vi "Begin map measurement.vi"(8 "Sweep down\ntime [ms]":dbl=500.0 format="%#_13g", 9 "VID control":T4 {"Multip" items=["1"=1, "2"=2, "3"=3, "4"=4, "6"=6, "8"=8, "9"=9]; "AMC" items=["9"=9, "12"=12]}, 10 "Map parameters":T2={"B_start[T]"=0.0, "B_End[T]"=0.0, "B_rate [mT/s]"=0.0, "F_start[GHz]"=0.0, "F_end[GHz]"=0.0, "Sampling rate"=0, "Tmp [K]"=0.0, "Wait[min]"=0.0, "Points"=0, "Display signal"=enum."Phi", "Signal treat"=enum."None", "Sweep [s]"=2.0} {"Sampling rate" items=["117 ks/S"=9, "58.6 kS/s"=10, "29.3 kS/s"=11, "14.6 kS/s"=12, "7.32 kS/s"=13, "3.66 kS/s"=14, "1.83 kS/s"=15]}, 11 "Referencies in":T1) -> (0 "error out":errorcluster)   [LabVIEW 2022 SP3]
uses:
  Datatypes/THz parameters.ctl
  Datatypes/Map parameters.ctl
  Subsystem modules/Lock-in module/ctl/OSC sampling rate.ctl
  Subsystem modules/Messenger service/Data types/Messenger referencies.ctl
  Subsystem modules/Lock-in module/ctl/MFLI_message for module.ctl
  Subsystem modules/Lock-in module/ctl/MFLI_command enum.ctl
  Subsystem modules/THz module/ctl/THz Message for module.ctl
  Subsystem modules/THz module/ctl/THz commands enum.ctl
  Subsystem modules/THz module/ctl/THz sweep parameters.ctl
  Subsystem modules/Magnet module/ctl/MSG to magnet.ctl
  Subsystem modules/Magnet module/ctl/Magnet Orders.ctl
  Subsystem modules/Magnet module/ctl/SetField data.ctl
  Subsystem modules/Magnet module/ctl/Magnet mode public.ctl
  Subsystem modules/Lock-in module/ctl/Mode.ctl
  Subsystem modules/Lock-in module/Lock-in module.lvlib
  Subsystem modules/THz module/THz source modeule.lvlib
  Subsystem modules/Magnet module/Magnet module.lvlib
  Subsystem modules/Messenger service/MessengerLib.lvlib
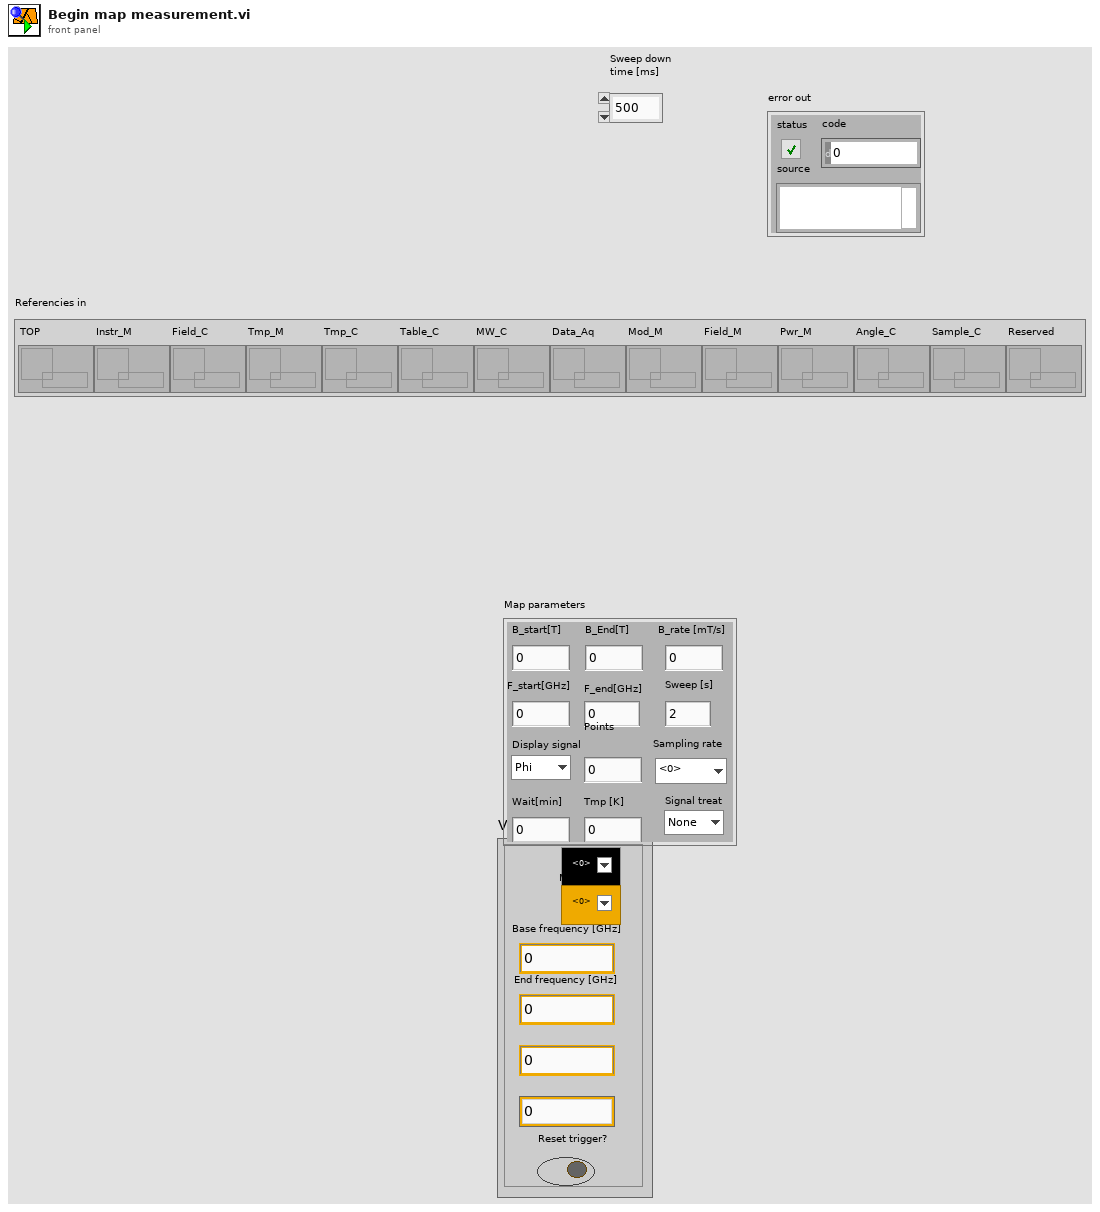
[diagram p1: front panel]
types:
  T1 = typedef "MessengerLib.lvlib/Messenger referencies.ctl" = cluster{"TOP":refnum<queue>, "Instr_M":refnum<queue>, "Field_C":refnum<queue>, "Tmp_M":refnum<queue>, "Tmp_C":refnum<queue>, "Table_C":refnum<queue>, "MW_C":refnum<queue>, "Data_Aq":refnum<queue>, "Mod_M":refnum<queue>, "Field_M":refnum<queue>, "Pwr_M":refnum<queue>, "Angle_C":refnum<queue>, "Sample_C":refnum<queue>, "Reserved":refnum<queue>}
  T2 = typedef "Map parameters.ctl" = cluster{"B_start[T]":dbl, "B_End[T]":dbl, "B_rate [mT/s]":dbl, "F_start[GHz]":dbl, "F_end[GHz]":dbl, "Sampling rate":T3, "Tmp [K]":dbl, "Wait[min]":dbl, "Points":u32, "Display signal":enum16{"X", "Y", "R", "Phi"}, "Signal treat":enum16{"None", "Unity norm", "Mean norm", "Standardization"}, "Sweep [s]":dbl}
  T3 = typedef "OSC sampling rate.ctl" = u16
  T4 = typedef "THz parameters.ctl" = cluster{"AMC":u16, "Multip":u16, "Base frequency [GHz]":dbl, "End frequency [GHz]":dbl, "Im frequency [MHz]":dbl, "Sweep up [ms]":dbl, "Reset trigger?":bool}
  T5 = typedef "Magnet module.lvlib/MSG to magnet.ctl" = cluster{"Command":T6, "Data":variant}
  T6 = typedef "Magnet module.lvlib/Magnet Orders.ctl" = enum16{"Ignore", "Connect", "Update", "Switch mode", "Set field", "Stop ramping", "Equalize output", "Zero output", "Flip polarity", "Blackout", "Set timer", "Eval temperatures", "Disconnect"}
  T7 = typedef "Lock-in module.lvlib/Mode.ctl" = enum16{"None", "Point", "Scope", "Both", "DAQ"}
  T8 = typedef "Magnet module.lvlib/SetField data.ctl" = cluster{"Field [T]":dbl, "Ramp [T/s]":dbl, "Custom Ramp?":bool, "Mode":T9}
  T9 = typedef "Magnet module.lvlib/Magnet mode public.ctl" = enum16{"Persistant", "Ramping"}
  T10 = typedef "THz source modeule.lvlib/THz sweep parameters.ctl" = cluster{"Start [GHz]":dbl, "End [GHz] ":dbl, "Sweep up\ntime [ms]":dbl, "Sweep down\ntime [ms]":dbl, "Intermidiate [MHz]":dbl, "Reset trigger":bool}
  T11 = typedef "THz source modeule.lvlib/THz Message for module.ctl" = cluster{"Command":T12, "Data":variant}
  T12 = typedef "THz source modeule.lvlib/THz commands enum.ctl" = enum16{"Ignore", "Connect", "Update", "Set parameters", "Disconnect", "End"}
  T13 = typedef "Lock-in module.lvlib/MFLI_message for module.ctl" = cluster{"Command":T14, "Data":variant}
  T14 = typedef "Lock-in module.lvlib/MFLI_command enum.ctl" = enum16{"Initialize", "Update", "Set parameters", "Set module", "Set individual parameters", "Get point", "Get array", "Disconnect", "End", "Ignore"}
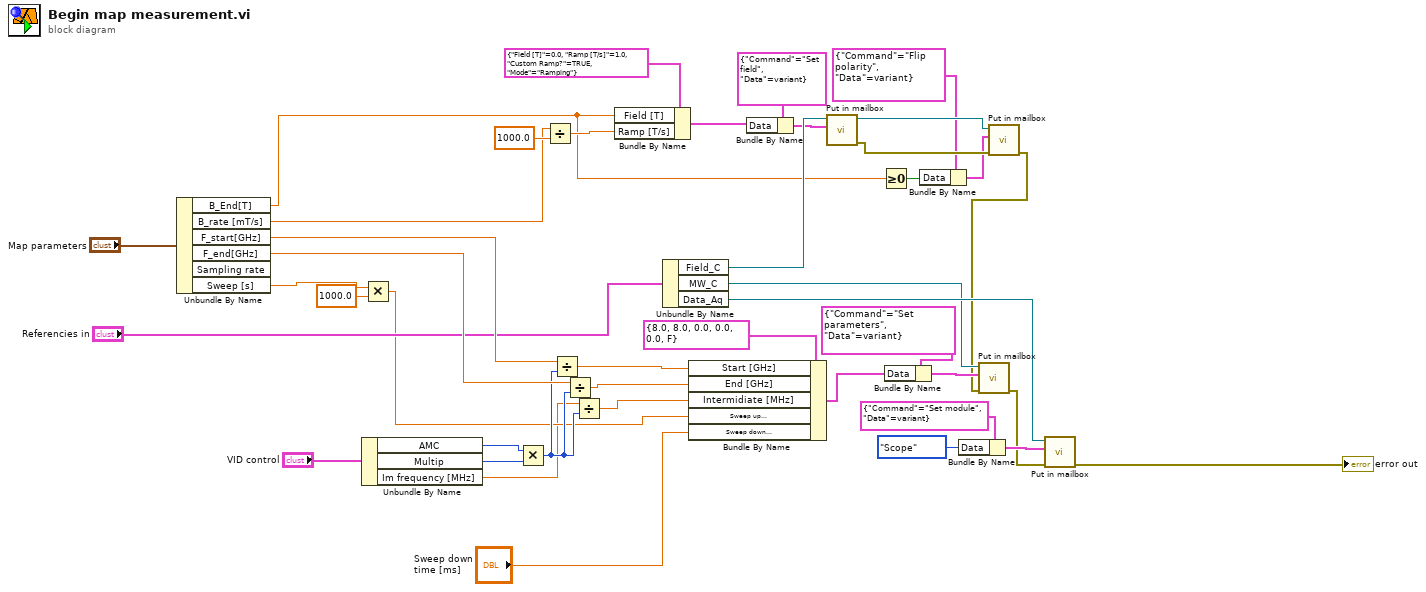
[diagram p0: block diagram]
diagram:
  n1 = Unbundle By Name("Map parameters") -> ("B_End[T]"=w2:dbl, "B_rate [mT/s]"=w31:dbl, "F_start[GHz]"=w41:dbl, "F_end[GHz]"=w42:dbl, "Sweep [s]"=w10:dbl)  [unwired: 1 out]
  n2 = Unbundle By Name("VID control") -> ("AMC"=w24:u16, "Multip"=w25:u16, "Im frequency [MHz]"=w1:dbl)
  n3 = Multiply(x=w10, y=1000.0) -> (x*y=w11:dbl)
  n4 = Multiply(x=w24, y=w25) -> (x*y=w13:u16)
  n5 = Divide(x=w31, y=1000.0) -> (x/y=w39:dbl)
  n6 = Divide(x=w41, y=w13) -> (x/y=w19:dbl)
  n7 = Divide(x=w42, y=w13) -> (x/y=w20:dbl)
  n8 = Divide(x=w1, y=w13) -> (x/y=w23:dbl)
  n9 = Bundle By Name(cluster=T8 {"Field [T]"=0.0, "Ramp [T/s]"=1.0, "Custom Ramp?"=TRUE, "Mode"=enum."Ramping"} ("Set Field"), "Field [T]"=w2, "Ramp [T/s]"=w39) -> (w15:T8)
  n10 = Unbundle By Name("Referencies in") -> ("Field_C"=w17:refnum<queue>, "MW_C"=w18:refnum<queue>, "Data_Aq"=w35:refnum<queue>)
  n11 = Bundle By Name(cluster=T10 {"Start [GHz]"=8.0, "End [GHz] "=8.0, "Sweep up\ntime [ms]"=0.0, "Sweep down\ntime [ms]"=0.0, "Intermidiate [MHz]"=0.0, "Reset trigger"=FALSE} ("Sweep parameters"), "Start [GHz]"=w19, "End [GHz]"=w20, "Intermidiate [MHz]"=w23, "Sweep up\ntime [ms]"=w11, "Sweep down\ntime [ms]"="Sweep down\ntime [ms]") -> (w21:T10)
  n12 = Bundle By Name(cluster=T5 {"Command"=enum."Set field", "Data"=variant} ("MSG to magnet"), "Data"=w15) -> (w16:T5)
  n13 = call "Put in mailbox.vi"("Message"=w16, "Queue in"=w17) -> ("error out"=w6:errorcluster, "Queue out"=w7:refnum<queue>)  [unwired: 7 in, 1 out]
  n14 = Greater Or Equal To 0?(x=w2) -> (x >= 0?=w3:bool)
  n15 = Bundle By Name(cluster=T11 {"Command"=enum."Set parameters", "Data"=variant} ("Incoming msg"), "Data"=w21) -> (w22:T11)
  n16 = Bundle By Name(cluster=T5 {"Command"=enum."Flip polarity", "Data"=variant} ("MSG to magnet"), "Data"=w3) -> (w4:T5)
  n17 = Bundle By Name(cluster=T13 {"Command"=enum."Set module", "Data"=variant} ("MSG for  ACQ"), "Data"=Mode."Scope" ("Mode")) -> (w37:T13)
  n18 = call "Put in mailbox.vi"("error in (no error)"=w6, "Message"=w4, "Queue in"=w7) -> ("error out"=w8:errorcluster)  [unwired: 6 in, 2 out]
  n19 = call "Put in mailbox.vi"("error in (no error)"=w8, "Message"=w22, "Queue in"=w18) -> ("error out"=w36:errorcluster)  [unwired: 6 in, 2 out]
  n20 = call "Put in mailbox.vi"("error in (no error)"=w36, "Message"=w37, "Queue in"=w35) -> ("error out"=→"error out":errorcluster)  [unwired: 6 in, 2 out]
